vi "RxBfrPkt - Handle Ping Pong Buffer.vi"(6 "Ext Buffer?":bool, 8 "error in (no error)":errorcluster, 11 "Node Ptr":T1 format="%.0x") -> (0 "error out":errorcluster, 3 "Node Ptr out":T1 format="%.0x")   [LabVIEW 2019, in "UDP-Custom-Device System Explorer.lvlib"]
uses:
  UDP-Custom-Device System Explorer.lvlib
  <vilib>/NI VeriStand/Custom Device API/Custom Device Item Ref.ctl
  <vilib>/NI VeriStand/Custom Device API/Custom Device Channel.ctl
  <vilib>/NI VeriStand/Custom Device API/Custom Device Channel Type.ctl
  Property Accessors/Buffered Data Packet.lvlib
  <vilib>/NI VeriStand/Custom Device API/Custom Device API.lvlib
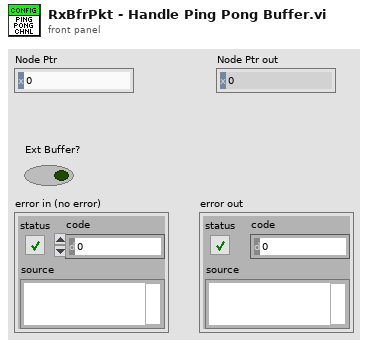
[diagram p1: front panel]
types:
  T1 = typedef "Custom Device API.lvlib/Custom Device Item Ref.ctl" = u64
  T2 = typedef "Custom Device API.lvlib/Custom Device Channel Type.ctl" = enum16{"Input", "Output"}
  T3 = typedef "Custom Device API.lvlib/Custom Device Channel.ctl" = cluster{"Type":T2, "Units":string, "Default Value":dbl, "Faultable":bool, "Scalable":bool}
  T4 = typedef "UDP-Custom-Device Shared.lvlib/Shared - Receive Buffer Options.ctl" = enum16{"Static Buffer", "Circular Buffer", "Circular Buffer + Size", "Internal Cache", "Internal Cache + Size", "Ping Pong", "Ping Pong + Size"}
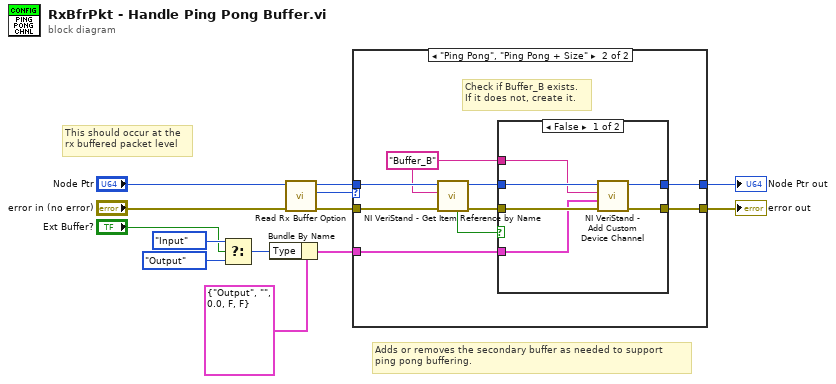
[diagram p0: block diagram]
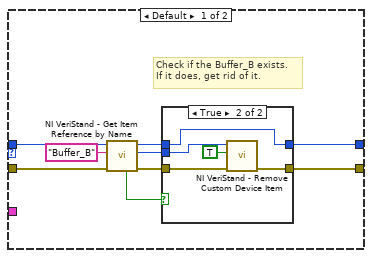
[diagram p2: hidden frame]
diagram:
  # "Adds or removes the secondary buffer as needed to support\nping pong buffering."
  # "This should occur at the\nrx buffered packet level"
  n1 = Select(t=Custom_Device_Channel_Type."Input" ("Type"), s="Ext Buffer?", f=Custom_Device_Channel_Type."Output" ("Type")) -> (s? t:f=w4:T2)
  n2 = Bundle By Name(cluster=T3 {"Type"=enum."Output", "Units"="", "Default Value"=0.0, "Faultable"=FALSE, "Scalable"=FALSE} ("Channel"), "Type"=w4) -> (w1:T3)
  n3 = call "Read Rx Buffer Option.vi"("error in (no error)"="error in (no error)", "Node Ptr"="Node Ptr") -> ("error out"=w9:errorcluster, "Buffer Option"=w11:T4, "Node Ptr out"=w10:T1)  [unwired: 7 in]
  n4 = case shown="\"Ping Pong\", \"Ping Pong + Size\"" w11 {
    tunnel: w10 -> [w22 w38]
    tunnel: w9 -> [w21 w37]
    tunnel: [w15 w35] -> w8
    tunnel: [w14 w32] -> w7
    tunnel: w1 -> [_ w31]
    frame Default {
      # "Check if the Buffer_B exists.\nIf it does, get rid of it."
      n5 = call <vilib>:"NI VeriStand - Get Item Reference by Name.vi"("error in (no error)"=w21, "Item Name"="Buffer_B", "Parent Ref in"=w22) -> ("error out"=w18:errorcluster, "Item Ref"=w17:T1, "Parent Ref out"=w16:T1, "Found"=w19:bool)  [unwired: 5 in]
      n6 = case shown="True" w19 {
        tunnel: w18 -> [w24 w28]
        tunnel: w17 -> [_ w29]
        tunnel: w16 -> [w23 w25]
        tunnel: [w24 w26] -> w15
        tunnel: [w23 w25] -> w14
        frame False {
        }
        frame True {
          n7 = call <vilib>:"NI VeriStand - Remove Custom Device Item.vi"("error in (no error)"=w28, "Force Delete (F)"=TRUE, "Item Ref in"=w29) -> ("error out"=w26:errorcluster)  [unwired: 7 in, 1 out]
        }
      }
    }
    frame "Ping Pong", "Ping Pong + Size" {
      w30 = "Buffer_B" ("Item Name")
      # "Check if Buffer_B exists.\nIf it does not, create it."
      n8 = call <vilib>:"NI VeriStand - Get Item Reference by Name.vi"("error in (no error)"=w37, "Item Name"=w30, "Parent Ref in"=w38) -> ("error out"=w34:errorcluster, "Parent Ref out"=w33:T1, "Found"=w36:bool)  [unwired: 5 in, 1 out]
      n9 = case shown="False" w36 {
        tunnel: [w42 w45] -> w35
        tunnel: w34 -> [w43 w45]
        tunnel: w33 -> [w44 w46]
        tunnel: [w41 w46] -> w32
        tunnel: w31 -> [w39 _]
        tunnel: w30 -> [w40 _]
        frame False {
          n10 = call <vilib>:"NI VeriStand - Add Custom Device Channel.vi"("error in (no error)"=w43, "Channel"=w39, "Channel Name"=w40, "Parent Ref in"=w44) -> ("error out"=w42:errorcluster, "Parent Ref out"=w41:T1)  [unwired: 4 in, 2 out]
        }
        frame True {
        }
      }
    }
  }
  "error out" <- w8
  "Node Ptr out" <- w7
